vi "Suite.vi"(8 "error in (no error)":errorcluster, 10 "LUnit Test Suite in":refnum<class "Test Suite.lvclass">, 11 "Parameterized Test Case In":refnum<class "Parameterized Test Case.lvclass">) -> (0 "error out":errorcluster, 2 "LUnit Test Suite Out":refnum<class "Test Suite.lvclass">, 3 "Parameterized Test Case Out":refnum<class "Parameterized Test Case.lvclass">)   [LabVIEW 2020, in "Parameterized Test Case.lvclass"]
doc: "Factory method to generate a Test Suite object for the test case class.\nThe Test Suite input is used as a collecting parameter to which the test case methods are appended. This can be useful when using custom test suite classes."
uses:
  Parameterized Test Case.lvclass
  <vilib>/Astemes/LUnit/Test Suite.lvclass
  C:/Program Files (x86)/National Instruments/LabVIEW 2020/vi.lib/Astemes/LUnit/LUnit Runnable.lvclass
  Parameterized Test Suite/Parameterized Test Suite.lvclass
  C:/Program Files (x86)/National Instruments/LabVIEW 2020/vi.lib/Astemes/LUnit/Test Suite.lvclass
  Parameter/Parameter.lvclass
  Parameterized Test Case.lvclass/Parameterized Test Case.ctl
  C:/git/astemes-lunit-parameterized-test/source/Parameterized Test Suite/Parameterized Test Suite.lvclass
  C:/Program Files (x86)/National Instruments/LabVIEW 2020/vi.lib/Astemes/LUnit/Test Case.lvclass
  C:/git/astemes-lunit-parameterized-test/source/Parameterized Test Case/Parameterized Test Case.lvclass
  C:/git/astemes-lunit-parameterized-test/source/Parameter/Parameter.lvclass
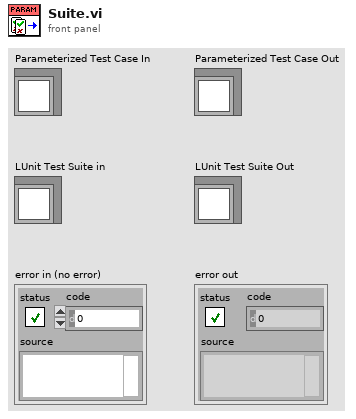
[diagram p1: front panel]
types:
  T1 = cluster{"Name":string, "Parameters":refnum<class "Parameterized Test Case.lvclass">}[]
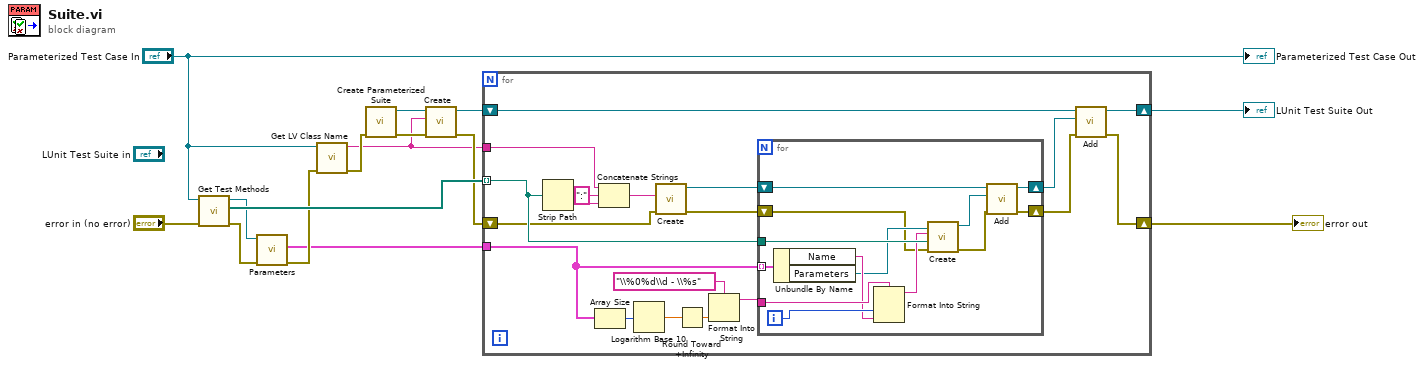
[diagram p0: block diagram]
diagram:
  n1 = call "Get Test Methods.vi"("error in (no error)"="error in (no error)", "Parameterized Test Case in"="Parameterized Test Case In") -> ("error out"=w3:errorcluster, "Array"=w10:path[], "Parameterized Test Case out"=w4:refnum<class "Parameterized Test Case.lvclass">)  [unwired: 7 in]
  n2 = call-dynamic "Parameters.vi"("error in (no error)"=w3, "Parameterized Test Case In"=w4) -> ("error out"=w2:errorcluster, "Parameters"=w1:T1)  [unwired: 8 in]
  n3 = call <vilib>:"Get LV Class Name.vi"("error in (no error)"=w2, "object"="Parameterized Test Case In") -> ("error out"=w12:errorcluster, "class name"=w5:string)  [unwired: 8 in]
  n4 = call "Create Parameterized Suite.vi"("error in (no error)"=w12) -> ("error out"=w15:errorcluster, "Parameterized Test Suite"=w14:refnum<class "Parameterized Test Suite.lvclass">)  [unwired: 9 in]
  n5 = call <vilib>:"Create.vi"("error in (no error)"=w15, "Suite Name"=w5, "LUnit Test Suite in"=w14) -> ("error out"=w8:errorcluster, "LUnit Test Suite Out"=w11:refnum<class "Parameterized Test Suite.lvclass">)  [unwired: 7 in]
  n6 = for {
    shift-right: [w24] -> w9
    shift-left: w11 -> [w25]
    tunnel: w10 -> [w34] mode=indexing
    shift-right: [w23] -> w6
    shift-left: w8 -> [w16]
    tunnel: w5 -> [w21]
    tunnel: w1 -> [w17]
    n7 = Strip Path(path=w34) -> (name=w33:string)  [unwired: 1 out]
    n8 = Array Size(array=w17) -> (size(s)=w29:i32)
    n9 = Concatenate Strings(w21, ":" ("string"), w33) -> (w22:string)
    n10 = Logarithm Base 10(1:w29) -> (0:w31:dbl)
    n11 = call <vilib>:"Create.vi"("error in (no error)"=w16, "Suite Name"=w22) -> ("error out"=w19:errorcluster, "LUnit Test Suite Out"=w27:refnum<class "Test Suite.lvclass">)  [unwired: 8 in]
    n12 = Round Toward +Infinity(x=w31) -> (ceil(x): smallest int >= x=w30:dbl)
    n13 = Format Into String(format string="\\%0%d\\d - \\%s", w30) -> (resulting string=w28:string)  [unwired: 2 in, 1 out]
    n14 = for {
      tunnel: w34 -> [w45]
      shift-right: [w46] -> w26
      shift-left: w27 -> [w47]
      tunnel: w17 -> [w44] mode=indexing
      tunnel: w28 -> [w42]
      shift-right: [w35] -> w18
      shift-left: w19 -> [w36]
      i -> [w43]
      n15 = Unbundle By Name(w44) -> ("Name"=w41:string, "Parameters"=w38:refnum<class "Parameterized Test Case.lvclass">)
      n16 = Format Into String(format string=w42, w43, w41) -> (resulting string=w40:string)  [unwired: 2 in, 1 out]
      n17 = call <vilib>:"Create.vi"("error in (no error)"=w36, "Test Method VI Path"=w45, "Name"=w40, "Parameterized Test Case"=w38) -> ("error out"=w37:errorcluster, "Parameter Out"=w39:refnum<class "Parameter.lvclass">)  [unwired: 6 in]
      n18 = call <vilib>:"Add.vi"("error in (no error)"=w37, "Runnable"=w39, "LUnit Test Suite In"=w47) -> ("error out"=w35:errorcluster, "LUnit Test Suite Out"=w46:refnum<class "Test Suite.lvclass">)  [unwired: 7 in]
    }
    n19 = call <vilib>:"Add.vi"("error in (no error)"=w18, "Runnable"=w26, "LUnit Test Suite In"=w25) -> ("error out"=w23:errorcluster, "LUnit Test Suite Out"=w24:refnum<class "Parameterized Test Suite.lvclass">)  [unwired: 7 in]
  }
  "error out" <- w6
  "LUnit Test Suite Out" <- w9
  "Parameterized Test Case Out" <- "Parameterized Test Case In"
